vi "Search.vi"() -> ()   [LabVIEW 2010]
uses:
  <vilib>/addons/database/_DB Variant To Data/Database Variant To Data.xnode
  <vilib>/addons/database/Connection.llb/DB Tools Open Connec (String).vi
  <vilib>/addons/database/Connection.llb/Conn Execute.vi
  <vilib>/addons/database/Recordset.llb/Rec Destroy - Connection.vi
  <vilib>/addons/database/NI_Database_API.lvlib
panel:
  out "exec_time":timestamp
  out "error in (no error)":errorcluster
  out "Database":string
  out "exp_id":i32
  out "submit_time":timestamp
  out "XML-String-in":string
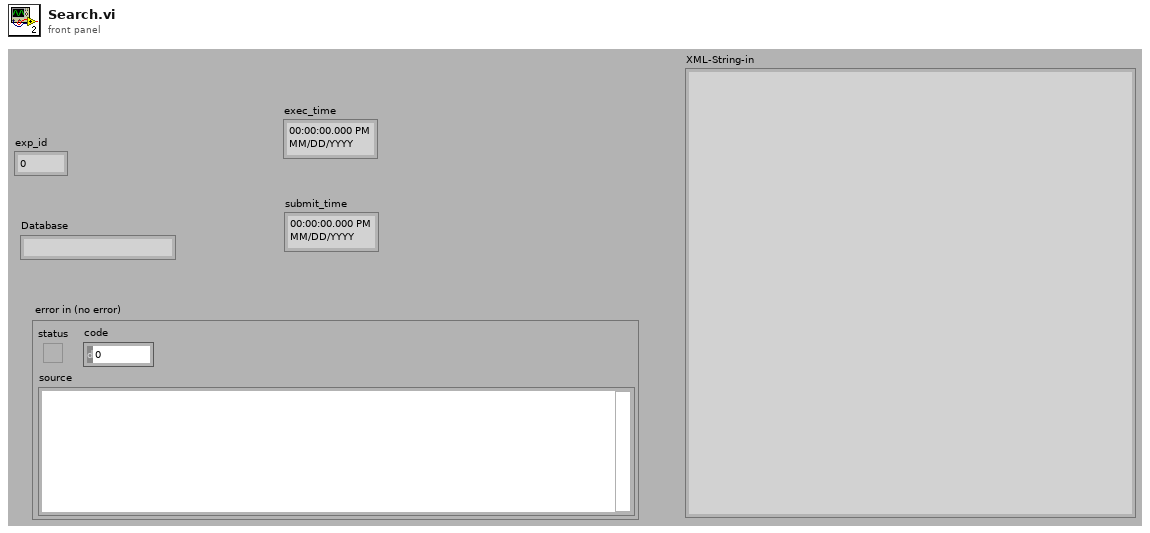
[diagram p1: front panel]
types:
  T1 = typedef "NI_Database_API.lvlib/Conn ObjectReference.ctl" = refnum<k1>
  T2 = typedef "NI_Database_API.lvlib/Rec ObjectReference.ctl" = refnum<k1>
  T3 = enum16{"Search", "Parse", "Run", "Assemble", "Set", ""}
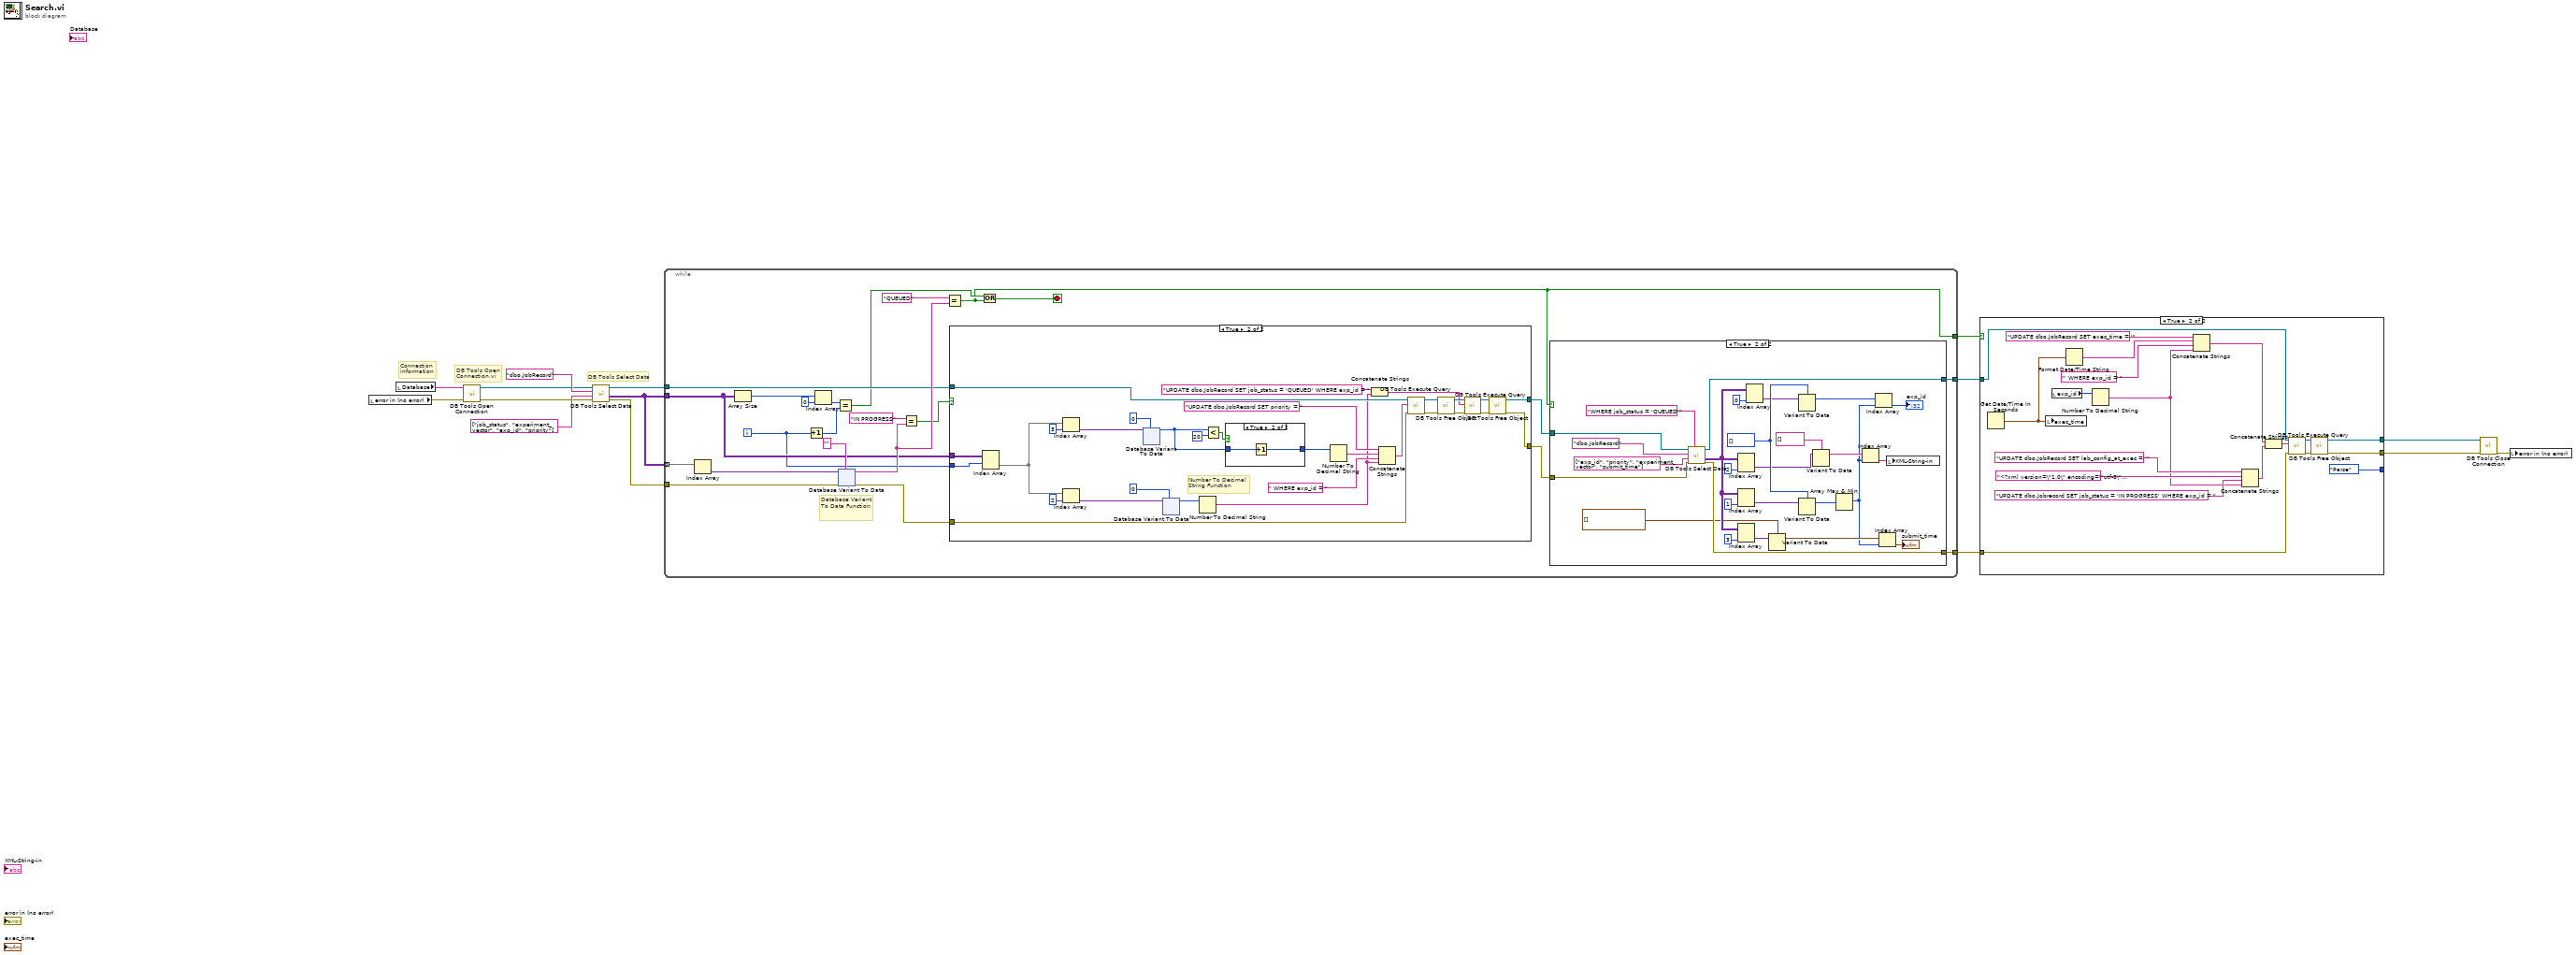
[diagram p0: block diagram]
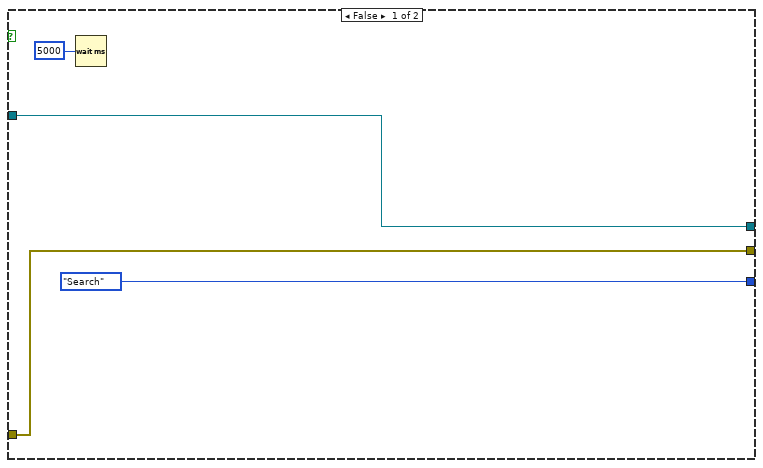
[diagram p2: hidden frame]
diagram:
  # "DB Tools Select Data"
  # "Connection \ninformation"
  # "DB Tools Open \nConnection.vi"
  n1 = local read "error in (no error)"() -> (w7:errorcluster)
  n2 = local read "Database"() -> (w11:string)
  n3 = call-poly <vilib>:"DB Tools Open Connection.vi"("error in (no error)"=w7, "connection information"=w11) -> ("error out"=w13:errorcluster, "connection reference"=w2:T1)  [unwired: 6 in]
  n4 = call <vilib>:"DB Tools Select Data.vi"("error in (no error)"=w13, "columns"=string[] ["job_status", "experiment_vector", "exp_id", "priority"], "table"="dbo.JobRecord", "connection reference"=w2) -> ("error out"=w6:errorcluster, "data"=w12:variant[][], "connection reference out"=w1:T1)  [unwired: 2 in]
  n5 = while {
    tunnel: w1 -> [w26]
    tunnel: [w30] -> w10
    tunnel: w12 -> [w35] mode=indexing
    tunnel: w12 -> [w24]
    tunnel: [w21] -> w3
    tunnel: w6 -> [w17]
    tunnel: [w18] -> w5
    i -> [w23]
    stop <- w20 stop-if-true
    # "Database Variant \nTo Data Function"
    n6 = Index Array(array=w35) -> (element=w36:variant)  [unwired: 1 in]
    n7 = Array Size(array=w24) -> (size(s)=w34:i32[])
    n8 = Increment(x=w23) -> (x+1=w31:i32)
    n9 = Index Array(array=w34, index=0) -> (element=w32:i32)
    n10 = Equal?(x=w32, y=w31) -> (x = y?=w22:bool)
    n11 = xnode "Database Variant To Data"("database variant"=w36, "error in"=w17, "type"="") -> ("data"=w29:string, "error out"=w16:errorcluster)
    n12 = Equal?(x="IN PROGRESS", y=w29) -> (x = y?=w27:bool)
    n13 = Equal?(x="QUEUED", y=w29) -> (x = y?=w21:bool)
    n14 = case shown="True" w27 {
      tunnel: w26 -> [w40 w60]
      tunnel: [w40 w56] -> w25
      tunnel: w24 -> [_ w71]
      tunnel: w23 -> [_ w41]
      tunnel: w16 -> [w39 w47]
      tunnel: [w39 w43] -> w19
      frame False {
      }
      frame True {
        # "Number To Decimal \nString Function"
        n15 = Index Array(array=w71, index (row)=w41) -> (element=w64:variant[])  [unwired: 1 in]
        n16 = Index Array(array=w64, index=3) -> (element=w69:variant)
        n17 = Index Array(array=w64, index=2) -> (element=w62:variant)
        n18 = xnode "Database Variant To Data"("database variant"=w69, "type"=0 ("index")) -> ("data"=w65:i32)  [unwired: 1 in, 1 out]
        n19 = xnode "Database Variant To Data"("database variant"=w62, "type"=0 ("index")) -> ("data"=w51:i32)  [unwired: 1 in, 1 out]
        n20 = Number To Decimal String(number=w51) -> (decimal integer string=w48:string)  [unwired: 1 in]
        n21 = Less?(x=w65, y=20) -> (x < y?=w66:bool)
        n22 = case shown="True" w66 {
          tunnel: w65 -> [w104 w106]
          tunnel: [w104 w105] -> w54
          frame False {
          }
          frame True {
            n23 = Increment(x=w106) -> (x+1=w105:i32)
          }
        }
        n24 = Number To Decimal String(number=w54) -> (decimal integer string=w53:string)  [unwired: 1 in]
        n25 = Concatenate Strings("UPDATE dbo.JobRecord SET job_status = 'QUEUED' WHERE exp_id = " ("string"), w48) -> (w42:string)
        n26 = Concatenate Strings("UPDATE dbo.JobRecord SET priority = " ("string"), w53, " WHERE exp_id = " ("string"), w48) -> (w50:string)
        n27 = call-poly <vilib>:"DB Tools Execute Query.vi"("error in (no error)"=w47, "SQL query"=w50, "connection reference"=w60) -> ("error out"=w46:errorcluster, "recordset reference"=w59:T2)  [unwired: 5 in]
        n28 = call-poly <vilib>:"DB Tools Free Object.vi"("error in (no error)"=w46, "recordset reference"=w59) -> ("error out"=w45:errorcluster, "connection reference"=w58:T1)  [unwired: 8 in]
        n29 = call-poly <vilib>:"DB Tools Execute Query.vi"("error in (no error)"=w45, "SQL query"=w42, "connection reference"=w58) -> ("error out"=w44:errorcluster, "recordset reference"=w57:T2)  [unwired: 5 in]
        n30 = call-poly <vilib>:"DB Tools Free Object.vi"("error in (no error)"=w44, "recordset reference"=w57) -> ("error out"=w43:errorcluster, "connection reference"=w56:T1)  [unwired: 8 in]
      }
    }
    n31 = Or(x=w22, y=w21) -> (x .or. y?=w20:bool)
    n32 = case shown="True" w21 {
      tunnel: w25 -> [w172 w190]
      tunnel: [w172 w189] -> w30
      tunnel: w19 -> [w171 w184]
      tunnel: [w171 w183] -> w18
      frame False {
      }
      frame True {
        w197 = i32[] [] ("Array")
        n33 = call <vilib>:"DB Tools Select Data.vi"("condition"="WHERE job_status = 'QUEUED'" ("optional clause"), "error in (no error)"=w184, "columns"=string[] ["exp_id", "priority", "experiment_vector", "submit_time"], "table"="dbo.JobRecord", "connection reference"=w190) -> ("error out"=w183:errorcluster, "data"=w179:variant[][], "connection reference out"=w189:T1)  [unwired: 1 in]
        n34 = Index Array(array=w179, index (col)=2 ("index (row)")) -> (element=w187:variant[])  [unwired: 1 in]
        n35 = Index Array(array=w179, index (col)=1 ("disabled index (col)")) -> (element=w194:variant[])  [unwired: 1 in]
        n36 = Index Array(array=w179, index (col)=3 ("disabled index (col)")) -> (element=w177:variant[])  [unwired: 1 in]
        n37 = Index Array(array=w179, index (col)=0 ("disabled index (col)")) -> (element=w196:variant[])  [unwired: 1 in]
        n38 = Variant To Data(Variant=w177, type=timestamp[] [] ("Array")) -> (data=w175:timestamp[])  [unwired: 1 in, 1 out]
        n39 = Variant To Data(Variant=w196, type=w197) -> (data=w199:i32[])  [unwired: 1 in, 1 out]
        n40 = Variant To Data(Variant=w194, type=w197) -> (data=w198:i32[])  [unwired: 1 in, 1 out]
        n41 = Variant To Data(Variant=w187, type=string[] [] ("Array")) -> (data=w186:string[])  [unwired: 1 in, 1 out]
        n42 = Array Max & Min(array=w198) -> (max index (indices)=w174:i32)  [unwired: 3 out]
        n43 = Index Array(array=w186, index=w174) -> (element=w185:string)
        n44 = Index Array(array=w199, index=w174) -> (element=→"exp_id":i32)
        n45 = Index Array(array=w175, index=w174) -> (element=→"submit_time":timestamp)
        n46 = local write "XML-String-in"(w185) -> ()
      }
    }
  }
  n47 = case shown="True" w3 {
    tunnel: [T3."Search" T3."Parse"] -> _
    tunnel: [w203 w215] -> w9
    tunnel: w10 -> [w203 w221]
    tunnel: w5 -> [w202 w220]
    tunnel: [w202 w218] -> w8
    frame False {
      n48 = Wait (ms)(milliseconds to wait=u32 5000 ("millisecond multiple")) -> ()  [unwired: 1 out]
    }
    frame True {
      n49 = Get Date/Time In Seconds() -> (seconds since 1Jan1904=w204:timestamp)
      n50 = local write "exec_time"(w204) -> ()
      n51 = local read "exp_id"() -> (w217:i32)
      n52 = Format Date/Time String(seconds (now)=w204) -> (date/time string=w213:string)  [unwired: 2 in]
      n53 = Number To Decimal String(number=w217) -> (decimal integer string=w208:string)  [unwired: 1 in]
      n54 = Concatenate Strings("UPDATE dbo.JobRecord SET exec_time = '", w213, "' WHERE exp_id = ", w208) -> (w207:string)
      n55 = Concatenate Strings("UPDATE dbo.JobRecord SET lab_config_at_exec = '" ("string"), "<?xml version=\"1.0\" encoding=\"utf-8\" standalone=\"no\" ?><!DOCTYPE labConfiguration SYSTEM \"http://web.mit.edu/weblab/xml/labConfiguration.dtd\"><labConfiguration lab=\"MIT ELVIS Weblab\" specversion=\"0.1\">'" ("string"), "UPDATE dbo.Jobrecord SET job_status = 'IN PROGRESS' WHERE exp_id = " ("string"), w208) -> (w206:string)
      n56 = Concatenate Strings(w207, w206) -> (w205:string)
      n57 = call-poly <vilib>:"DB Tools Execute Query.vi"("error in (no error)"=w220, "SQL query"=w205, "connection reference"=w221) -> ("error out"=w219:errorcluster, "recordset reference"=w216:T2)  [unwired: 5 in]
      n58 = call-poly <vilib>:"DB Tools Free Object.vi"("error in (no error)"=w219, "recordset reference"=w216) -> ("error out"=w218:errorcluster, "connection reference"=w215:T1)  [unwired: 8 in]
    }
  }
  n59 = call <vilib>:"DB Tools Close Connection.vi"("error in (no error)"=w8, "connection reference"=w9) -> ("error out"=w4:errorcluster)  [unwired: 5 in]
  n60 = local write "error in (no error)"(w4) -> ()
